vi "FlowPID2.vi"() -> ()   [LabVIEW 2017]
uses:
  BERTTA.dll
panel:
  out "lasttime":dbl
  out "timechange":dbl
  out "error":dbl
  out "errsum":dbl
  out "output2":dbl
  out "amount_out":dbl
  in  "flow_in":dbl
  out "Waveform Chart":dynamicdata(graph)
  in  "kd":dbl
  in  "ki":dbl=1e-05
  in  "kp":dbl=0.001
  in  "Setpoint":dbl=2000.0
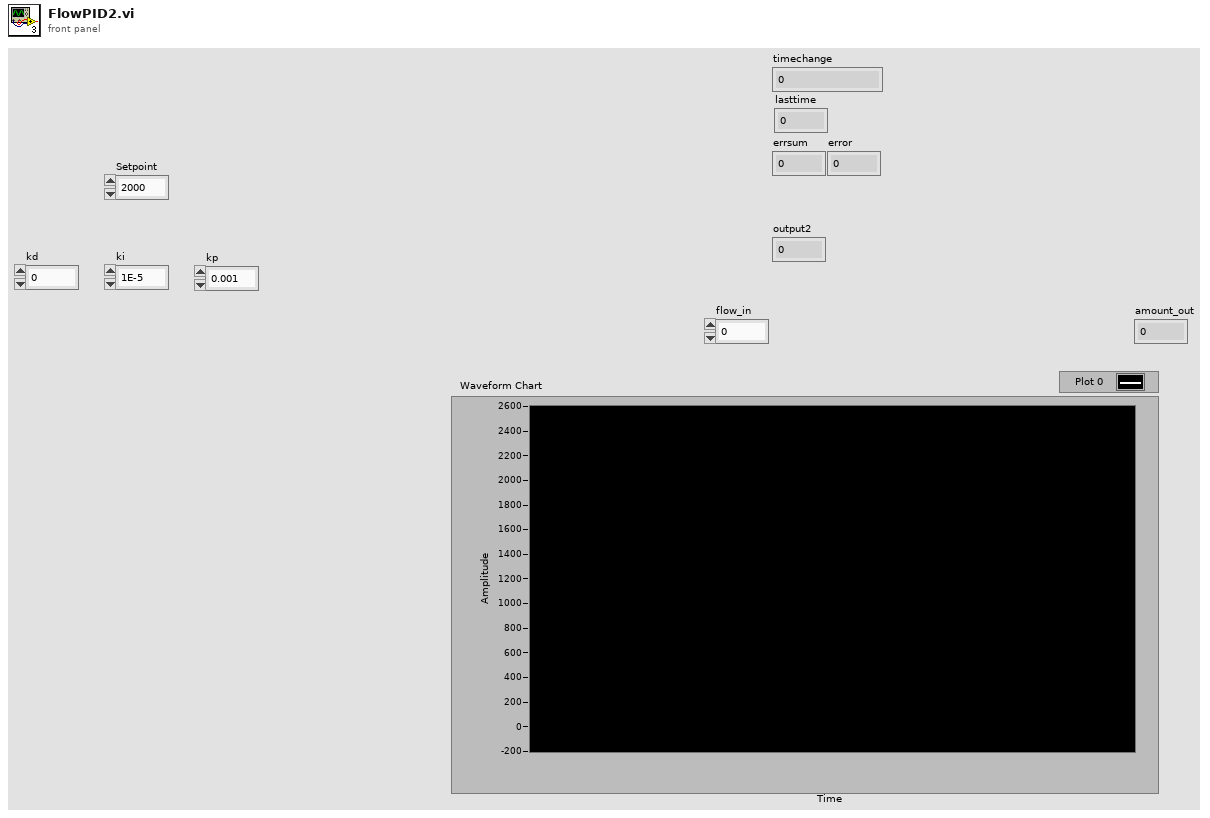
[diagram p1: front panel]
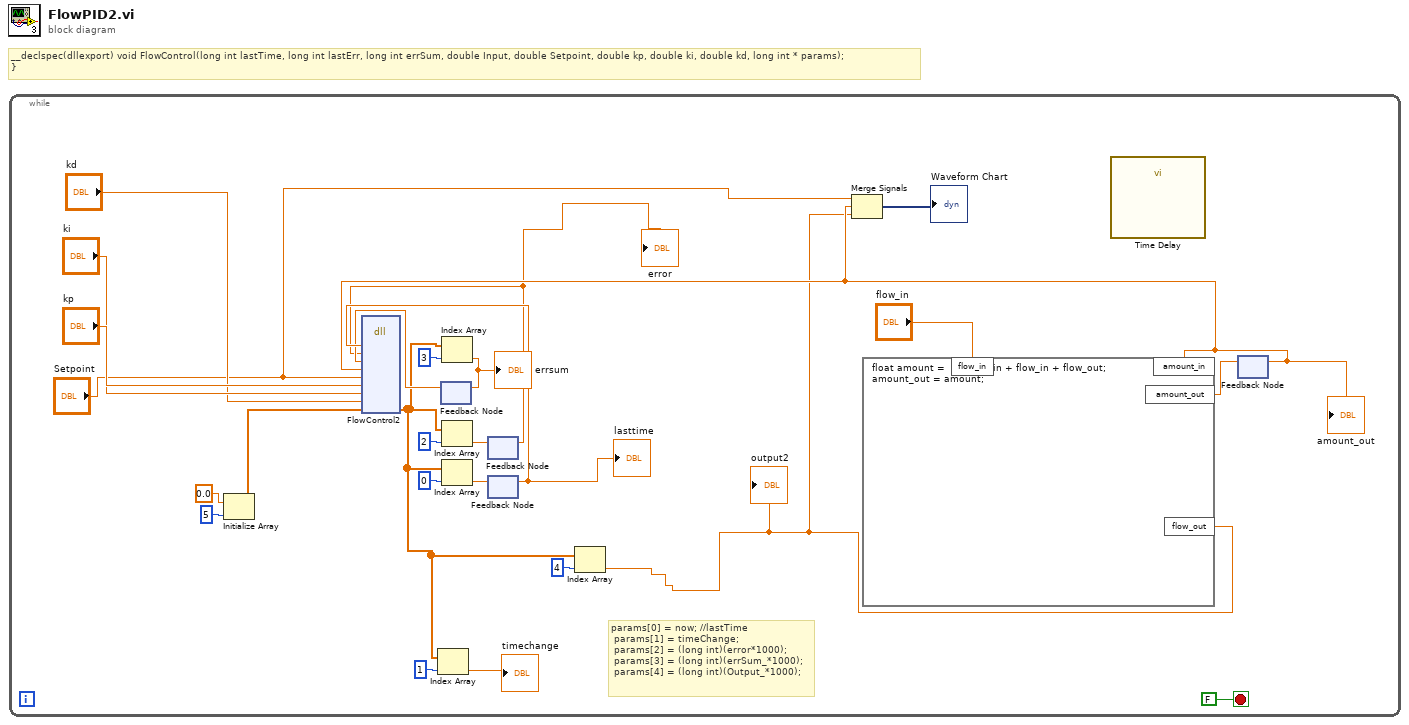
[diagram p0: block diagram]
diagram:
  # "__declspec(dllexport) void FlowControl(long int lastTime, long int lastErr, long int errSum, double Input, double Setpoint, double kp, double ki, double kd, long int * params);\n}"
  n1 = while {
    stop <- FALSE stop-if-true
    # "params[0] = now; //lastTime\n\tparams[1] = timeChange;\n\tparams[2] = (long int)(error*1000);\n\tparams[3] = (long int)(errSum_*1000);\n\tparams[4] = (long int)(Output_*1000);"
    n2 = Initialize Array(0.0 ("element"), 5 ("dimension size")) -> (w23:dbl[])
    n3 = feedback #1() -> (w10:dbl)  [unwired: 1 in]
    n4 = feedback #2() -> (w3:dbl)  [unwired: 1 in]
    "error" <- w3
    n5 = feedback #3() -> (w16:dbl)  [unwired: 1 in]
    "lasttime" <- w16
    n6 = call "Time Delay"() -> ()  [unwired: 11 in, 1 out]
    n7 = feedback #4() -> (w4:dbl)  [unwired: 1 in]
    "amount_out" <- w4
    n8 = dll-call lib="C:/Users/p3cn/OneDrive - Kemira Oyj/Documents/GitHub/Bertta/BERTTA/x64/Release/BERTTA.dll" fn="FlowControl2"("lastTime"=w16, "lastErr"=w3, "errSum"=w10, "Input"=w4, "Setpoint"="Setpoint", "kp"="kp", "ki"="ki", "kd"="kd", "PIDparams"=w23) -> ("PIDparams"=w1:dbl[])  [unwired: 12 in, 2 out]
    n9 = Index Array(array=w1, index=1) -> (element=→"timechange":dbl)
    n10 = Index Array(array=w1, index=3) -> (element=w11:dbl)
    "errsum" <- w11
    n11 = feedback-in #1(w11) -> ()
    n12 = Index Array(array=w1, index=2) -> (element=w13:dbl)
    n13 = Index Array(array=w1, index=0) -> (element=w17:dbl)
    n14 = feedback-in #2(w13) -> ()
    n15 = feedback-in #3(w17) -> ()
    n16 = Index Array(array=w1, index=4) -> (element=w2:dbl)
    "output2" <- w2
    n17 = Merge Signals("Setpoint", w4, w2) -> (→"Waveform Chart":dynamicdata)
    n18 = formula code="float amount =  amount_in + flow_in + flow_out;\namount_out = amount;"("flow_in"="flow_in", "amount_in"=w4, "flow_out"=w2) -> ("amount_out"=w7:dbl)
    n19 = feedback-in #4(w7) -> ()
  }
